vi "Returning Values By Reference Integer.vi"(8 "error in (no error)":errorcluster, 9 "sum":i32, 10 "y":i32, 11 "x":i32) -> (0 "error out":errorcluster, 1 "sum out":i32)   [LabVIEW 2009, in "LabVIEWWrapper_PassingDataSampleDLL.lvlib"]
doc: "void ReturningValuesByReference_Integer (int x, int y, int *sum);"
uses:
  LabVIEWWrapper_PassingDataSampleDLL.lvlib
  PassingDataSampleDLL.dll
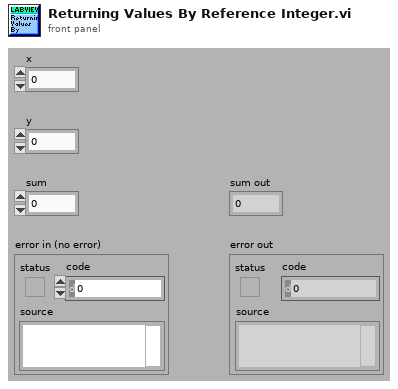
[diagram p1: front panel]
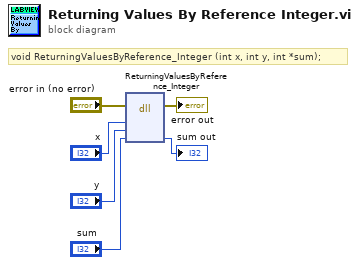
[diagram p0: block diagram]
diagram:
  # "void ReturningValuesByReference_Integer (int x, int y, int *sum);"
  n1 = dll-call lib="C:/My Dropbox/Systems Engineering Application/SDK/C Integration/LabVIEWWrapper/PassingDataSampleDLL.*" fn="ReturningValuesByReference_Integer"(error in="error in (no error)", "x"="x", "y"="y", "sum"="sum") -> (error out=→"error out":errorcluster, "sum"=→"sum out":i32)  [unwired: 5 in, 1 out]
